vi "Stepper Wait Till Steps Complete.vi"(8 "Error In":errorcluster, 11 "ChipKit Resource":T1={"COM Port"="", "Board Type"=enum."ChipKit uC32", "Connection Type"=enum."USB / Serial", "Baud Rate (115200)"=15, "Bytes Per Packet (15)"=15, "DI Port Num Pins"=0, "DO Port Num Pins"=0}) -> (0 "Error Out":errorcluster, 3 "ChipKit Resource":T1={"COM Port"="", "Board Type"=enum."ChipKit uC32", "Connection Type"=enum."USB / Serial", "Baud Rate (115200)"=15, "Bytes Per Packet (15)"=15, "DI Port Num Pins"=0, "DO Port Num Pins"=0})   [LabVIEW 2011, in "LabVIEW Interface for ChipKit.lvlib"]
doc: "This VI blocks and allows execution to continue after there are no further stepper commands in need of processing."
uses:
  LabVIEW Interface for ChipKit.lvlib
  Private/Type Defs/Chipkit Resource.ctl
  Private/Type Defs/Board Type.ctl
  Private/Type Defs/Connection Type.ctl
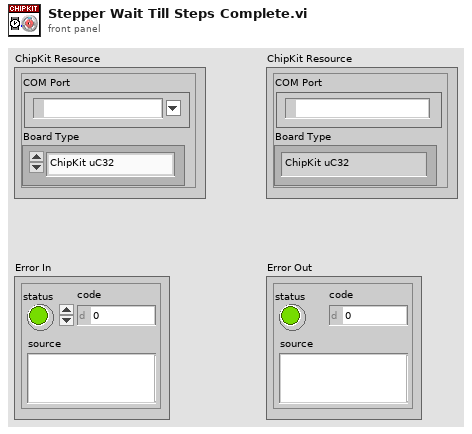
[diagram p1: front panel]
types:
  T1 = typedef "LabVIEW Interface for ChipKit.lvlib/Chipkit Resource.ctl" = cluster{"COM Port":refnum<visa-resource-name>, "Board Type":T2, "Connection Type":T3, "Baud Rate (115200)":u32, "Bytes Per Packet (15)":u32, "DI Port Num Pins":i32, "DO Port Num Pins":i32}
  T2 = typedef "LabVIEW Interface for ChipKit.lvlib/Board Type.ctl" = enum16{"ChipKit uC32", "ChipKit Uno32", "ChipKit Max32"}
  T3 = typedef "LabVIEW Interface for ChipKit.lvlib/Connection Type.ctl" = enum8{"USB / Serial", "XBEE", "BlueSmirf (Bluetooth)"}
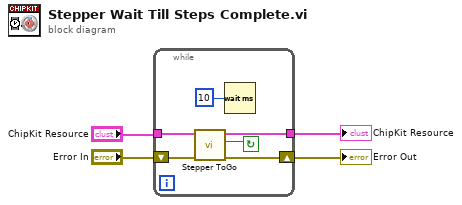
[diagram p0: block diagram]
diagram:
  n1 = while {
    tunnel: [w6] -> w1
    shift-right: [w7] -> w2
    shift-left: "Error In" -> [w8]
    tunnel: "ChipKit Resource" -> [w9]
    stop <- w5 continue-if-true
    n2 = call "Stepper ToGo.vi"("Error In"=w8, "ChipKit Resource"=w9) -> ("Error Out"=w7:errorcluster, "Steps Remaining?"=w5:bool, "ChipKit Resource"=w6:T1)  [unwired: 6 in, 1 out]
    n3 = Wait (ms)(milliseconds to wait=u32 10) -> ()  [unwired: 1 out]
  }
  "Error Out" <- w2
  "ChipKit Resource" <- w1
